vi "Init.vi"(8 "error in (no error)":errorcluster, 10 "Connection String":string, 11 "CameraDemo in":refnum<class "CameraDemo.lvclass">) -> (0 "error out":errorcluster, 3 "CameraDemo out":refnum<class "CameraDemo.lvclass">)   [LabVIEW 2020, in "CameraI2COUSB.lvlib" / "CameraDemo.lvclass"]
doc: "Inizialize camera object\n\n<b> ConnectionString:</b> String with parameters needed to connecting to camera. The parameters are separate by ::\nThe format is: <Vid>::<Pid>::<Device Index>::<Clock Rate>::<Provider Name>"
uses:
  CameraDemo.lvclass
  CameraDemo.lvclass/CameraDemo.ctl
  <vilib>/Utility/error.llb/Error Cluster From Error Code.vi
  <vilib>/ErrorRing/Error Ring.xnode
  Private/TypeDef/Init_Step.ctl
  Private/TypeDef/Init_FSMDate.ctl
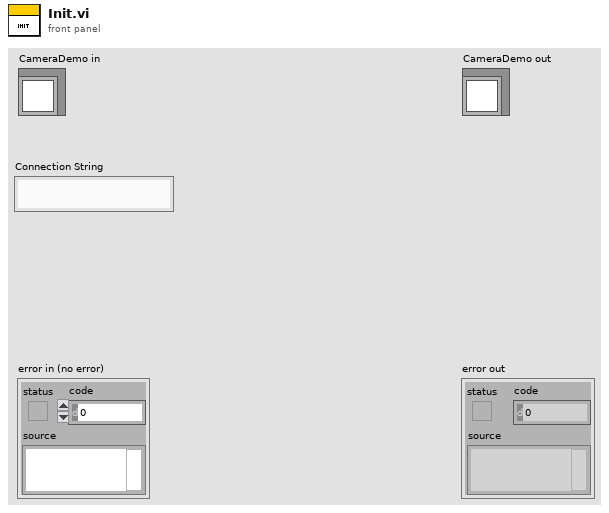
[diagram p1: front panel]
types:
  T1 = typedef "CameraI2COUSB.lvlib/CameraDemo.lvclass/Init_FSMDate.ctl" = cluster{"States":T2[], "PrjctItemRef":refnum<vi>}
  T2 = typedef "CameraI2COUSB.lvlib/CameraDemo.lvclass/Init_Step.ctl" = enum16{"Map Cmds to Registers", "Set Path Driver Info", "AcquireConnPrms", "CheckDriverFolder", "FindDriverClass", "LoadDriver"}
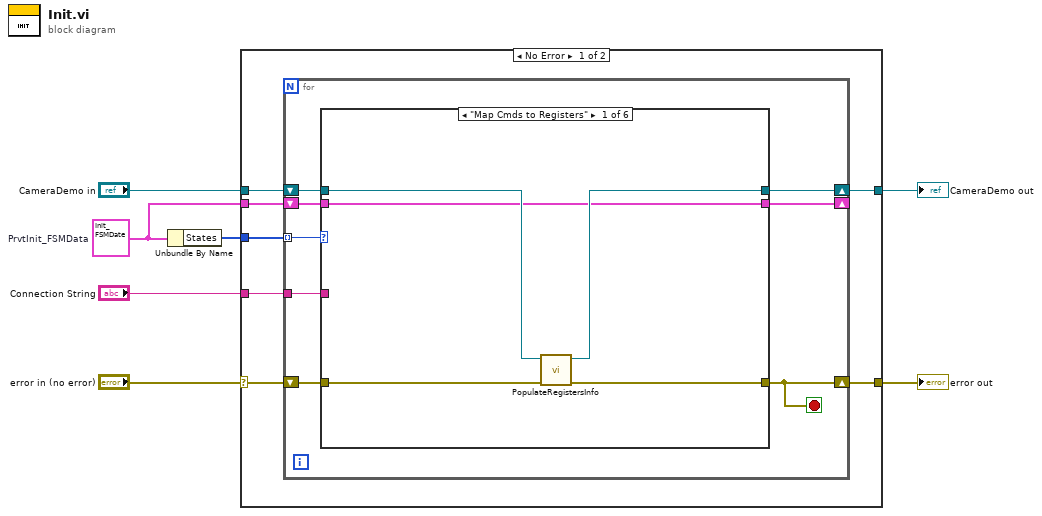
[diagram p0: block diagram]
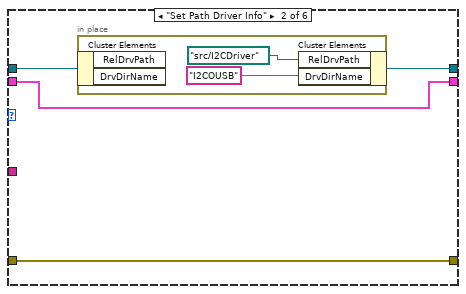
[diagram p2: hidden frame]
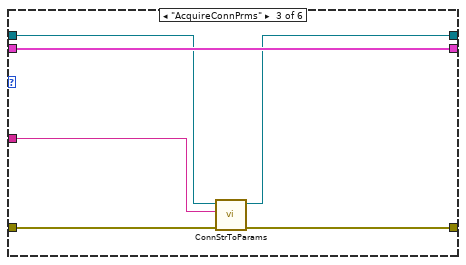
[diagram p3: hidden frame]
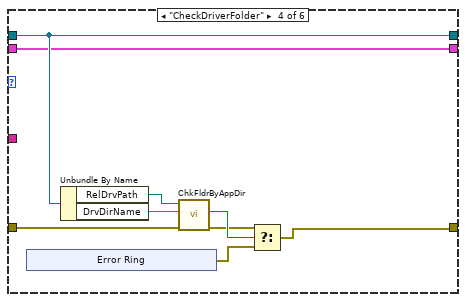
[diagram p4: hidden frame]
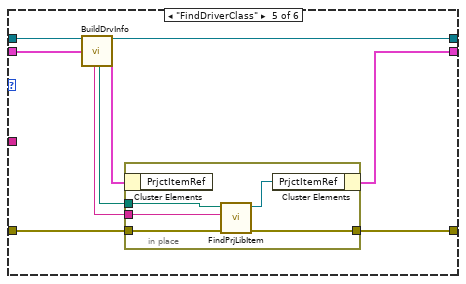
[diagram p5: hidden frame]
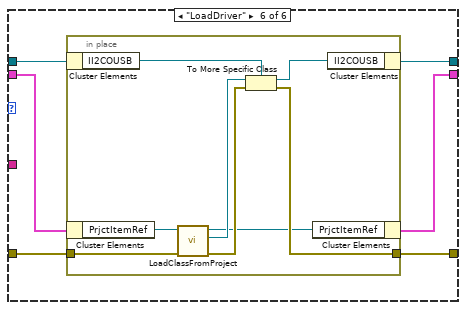
[diagram p6: hidden frame]
diagram:
  w6 = T1 {"States"=[enum."Map Cmds to Registers", enum."Set Path Driver Info", enum."CheckDriverFolder", enum."FindDriverClass", enum."LoadDriver"], "PrjctItemRef"=refnum}  # PrvtInit_FSMData
  n1 = Unbundle By Name(w6) -> ("States"=w7:T2[])
  n2 = case shown="No Error" "error in (no error)" {
    selector: "error in (no error)" -> [w11 w82]
    tunnel: [w8 w82] -> w1
    tunnel: [w13 w81] -> w5
    tunnel: "CameraDemo in" -> [w14 w81]
    tunnel: "Connection String" -> [w12 _]
    tunnel: w6 -> [w10 _]
    tunnel: w7 -> [w9 _]
    frame No Error {
      n3 = for {
        shift-right: [w19] -> w13
        shift-left: w14 -> [w20]
        tunnel: w12 -> [w22]
        shift-right: [w15] -> w8
        shift-left: w11 -> [w21]
        shift-right: [w17] -> _
        shift-left: w10 -> [w18]
        tunnel: w9 -> [w16] mode=indexing
        stop <- w15 stop-if-true
        n4 = case shown="\"Map Cmds to Registers\"" w16 {
          tunnel: w22 -> [_ _ w39 _ _ _]
          tunnel: w21 -> [w26 w29 w36 w48 w55 w72]
          tunnel: [w24 w29 w35 w44 w54 w69] -> w15
          tunnel: w20 -> [w27 w31 w37 w43 w59 w71]
          tunnel: [w25 w30 w34 w43 w58 w68] -> w19
          tunnel: w18 -> [w23 w28 w38 w42 w61 w70]
          tunnel: [w23 w28 w38 w42 w60 w67] -> w17
          frame "Map Cmds to Registers" {
            n5 = call "PopulateRegistersInfo.vi"("error in (no error)"=w26, "CameraDemo in"=w27) -> ("error out"=w24:errorcluster, "CameraDemo out"=w25:refnum<class "CameraDemo.lvclass">)  [unwired: 8 in]
          }
          frame "Set Path Driver Info" {
            n6 = in-place {
              n7 = in-place-cluster #1(w31) -> ()  [unwired: 2 out]
              n8 = in-place-cluster #1("RelDrvPath"=path "src/I2CDriver" ("Rel. Driver Path"), "DrvDirName"="I2COUSB" ("Folder Name")) -> (w30:refnum<class "CameraDemo.lvclass">)
            }
          }
          frame "AcquireConnPrms" {
            n9 = call "ConnStrToParams.vi"("error in (no error)"=w36, "Connection String"=w39, "CameraDemo in"=w37) -> ("error out"=w35:errorcluster, "CameraDemo out"=w34:refnum<class "CameraDemo.lvclass">)  [unwired: 7 in]
          }
          frame "CheckDriverFolder" {
            n10 = xnode "Error Ring"() -> ("error out"=w45:errorcluster)
            n11 = Unbundle By Name(w43) -> ("RelDrvPath"=w41:path, "DrvDirName"=w40:string)
            n12 = call "ChkFldrByAppDir.vi"("error in (no error)"=w48, "Folder Name"=w40, "Rel. Path"=w41) -> ("error out"=w46:errorcluster, "file or folder exists?"=w47:bool)  [unwired: 7 in]
            n13 = Select(t=w46, s=w47, f=w45) -> (s? t:f=w44:errorcluster)
          }
          frame "FindDriverClass" {
            n14 = call "BuildDrvInfo.vi"("CameraDemo in"=w59) -> ("CameraDemo out"=w58:refnum<class "CameraDemo.lvclass">, "Lib Path"=w57:path, "Class Name"=w56:string)  [unwired: 16 in]
            n15 = in-place {
              in-place-border: w57 -> [w65]
              in-place-border: w56 -> [w64]
              in-place-border: w55 -> [w63]
              in-place-border: [w62] -> w54
              n16 = in-place-cluster #2(w61) -> ()  [unwired: 1 out]
              n17 = call "FindPrjLibItem.vi"("error in (no error)"=w63, "Item Name"=w64, "Lib Path"=w65) -> ("error out"=w62:errorcluster, "ProjectItem Refnum"=w66:refnum<vi>)  [unwired: 7 in]
              n18 = in-place-cluster #2("PrjctItemRef"=w66) -> (w60:T1)
            }
          }
          frame "LoadDriver" {
            n19 = in-place {
              in-place-border: w72 -> [w79]
              in-place-border: [w75] -> w69
              n20 = in-place-cluster #3(w71) -> ("II2COUSB"=w80:refnum<class "II2COUSB.lvclass">)
              n21 = in-place-cluster #4(w70) -> ("PrjctItemRef"=w78:refnum<vi>)
              n22 = call "LoadClassFromProject.vi"("error in (no error)"=w79, "PrjctItemRef"=w78) -> ("error out"=w74:errorcluster, "object"=w77:refnum<class>, "PrjctItemRef"=w73:refnum<vi>)  [unwired: 7 in]
              n23 = To More Specific Class(target class=w80, reference=w77, error in=w74) -> (specific class reference=w76:refnum<class "II2COUSB.lvclass">, error out=w75:errorcluster)
              n24 = in-place-cluster #4("PrjctItemRef"=w73) -> (w67:T1)
              n25 = in-place-cluster #3("II2COUSB"=w76) -> (w68:refnum<class "CameraDemo.lvclass">)
            }
          }
        }
      }
    }
    frame Error {
    }
  }
  "error out" <- w1
  "CameraDemo out" <- w5
